vi "Local Variables.vi"() -> ()   [LabVIEW 2010]
panel:
  in  "루프 컨트롤":bool
  out "차트 2":dbl(graph)
  out "차트 1":dbl(graph)
  # "Off"
  # "On"
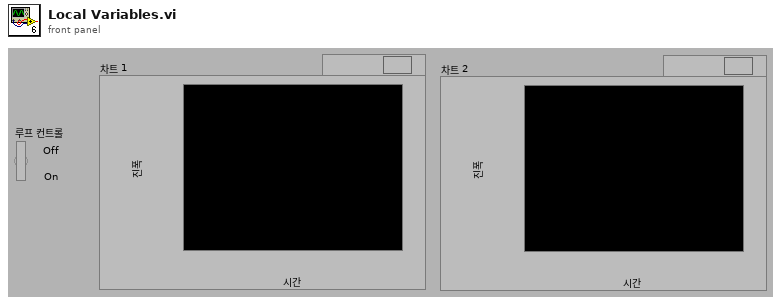
[diagram p1: front panel]
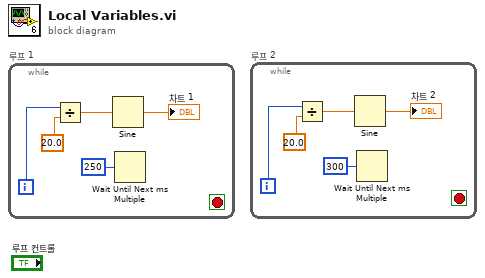
[diagram p0: block diagram]
diagram:
  n1 = while "루프 1" {
    i -> [w5]
    stop <- _ stop-if-true
    n2 = Divide(x=w5, y=20.0) -> (x/y=w3:dbl)
    n3 = Sine(x=w3) -> (sin(x)=→"차트 1":dbl)
    n4 = Wait Until Next ms Multiple(millisecond multiple=u32 250) -> ()  [unwired: 1 out]
  }
  n5 = while "루프 2" {
    i -> [w10]
    stop <- _ stop-if-true
    n6 = Divide(x=w10, y=20.0) -> (x/y=w8:dbl)
    n7 = Sine(x=w8) -> (sin(x)=→"차트 2":dbl)
    n8 = Wait Until Next ms Multiple(millisecond multiple=u32 300) -> ()  [unwired: 1 out]
  }
